vi "FTW-Test-JSON-Variants.vi"() -> ()   [LabVIEW 2018]
uses:
  69b651e3-3f07-4f5a-8146-147dca94f262.vi
  source/JSON/core/FTW-JSON-Core-EncodingFlags.vi
  source/Reflection/FTW-Reflection-Type.vi
  source/JSON/FTW-JSON-Parse.vi
  source/container/FTW-Container-GetFlattenedValue.vi
panel:
  out "variant":variant
  out "Values 2":cluster{"Variant":variant}
  out "Values":variant
  out "error out":errorcluster
  out "JSON String":string
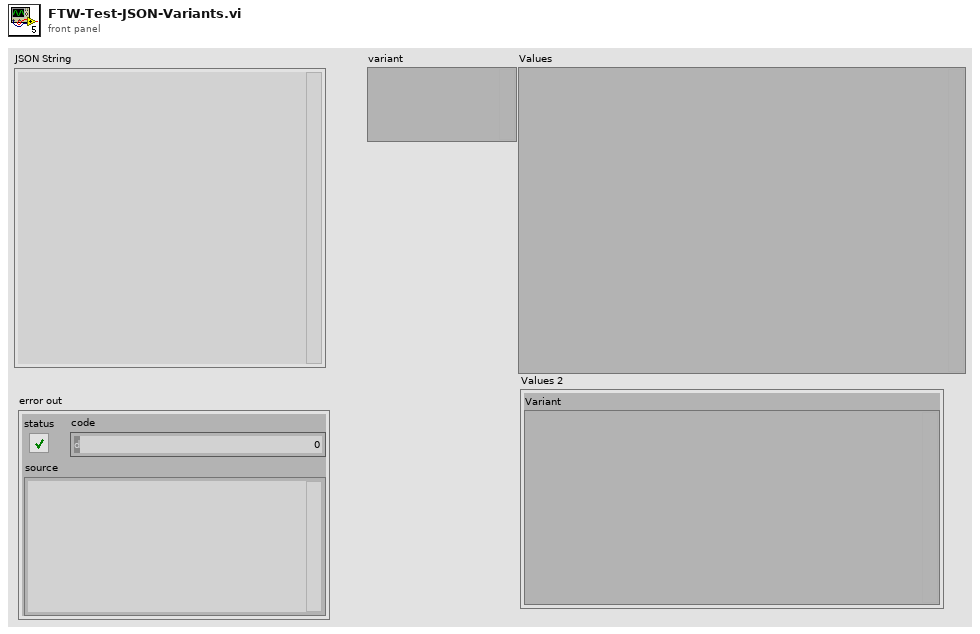
[diagram p1: front panel]
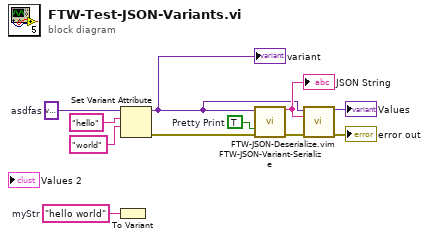
[diagram p0: block diagram]
diagram:
  w2 = variant  # asdfas
  w10 = TRUE  # Pretty Print
  w11 = "hello world"  # myStr
  n1 = To Variant(anything=w11) -> ()  [unwired: 1 out]
  n2 = Set Variant Attribute(Variant=w2, name="hello", value="world") -> (Variant out=w1:variant, error out=w3:errorcluster)  [unwired: 1 in, 1 out]
  "variant" <- w1
  n3 = call "FTW-JSON-Variant-Serialize.vi"("Variant"=w1, "Pretty Print"=w10, "error in"=w3) -> ("JSON String"=w7:string, "error out"=w6:errorcluster)  [unwired: 11 in]
  "JSON String" <- w7
  n4 = call "FTW-JSON-Deserialize.vim"("Type In"=w1, "JSON String"=w7, "error in"=w6) -> ("Type Out"=→"Values":variant, "error out"=→"error out":errorcluster)  [unwired: 11 in]
